vi "Teleop.vi"(10 "Match Info":T1={"Autonomous Elapsed Seconds"=0.0, "TeleOp Elapsed Seconds"=0.0, "Disabled Elapsed Seconds"=0.0, "Visited Autonomous"=FALSE, "Visited TeleOp"=FALSE, "Visited Disabled"=FALSE, "Autonomous Settings"={"Autonomous Style"=enum."Independent", "VI Refnum"=refnum}}, 11 "Call Context":T2) -> ()   [LabVIEW 2019]
doc: "This VI is called for each TeleOp packet received from the DS where the robot is not disabled. It is often used to read from the joysticks and update I/O or to update setpoints for timed control loops. It should complete and return within 20 milliseconds or it may miss DS packets."
uses:
  <vilib>/Rock Robotics/WPI/DriverStation/WPI_DriverStationDerivedRobotMode.ctl
  <vilib>/Rock Robotics/WPI/DriverStation/WPI_DriverStationMatch Info.ctl
  <vilib>/Rock Robotics/WPI/Solenoid/WPI_SolenoidValue.ctl
  <vilib>/Rock Robotics/WPI/ThirdParty/Phoenix-LabVIEW/Motor Controller/Controls/CTRE_Phoenix_MotorControl_ControlMode.ctl
  f70f45e1-7626-4a9c-a34c-83f61dc48ac5.vi
  <vilib>/Rock Robotics/WPI/Utilities/WPI_GetSetVariantRefNum.vi
  <vilib>/Rock Robotics/Network Tables/NT Write Boolean Array.vi
  <vilib>/Rock Robotics/Network Tables/NT Write Numeric Array.vi
  <vilib>/Rock Robotics/Network Tables/NT Read Boolean.vi
  <vilib>/Rock Robotics/Network Tables/NT Read Number.vi
  <vilib>/Rock Robotics/WPI/Solenoid/WPI_SolenoidSetEnum.vi
  <vilib>/Rock Robotics/Network Tables/NT Write Boolean.vi
panel:
  out "Sample Slider 0":dbl(slide) scale=0.0..5.0
  out "Sample Boolean 1":bool
  out "Sample Boolean 0":bool
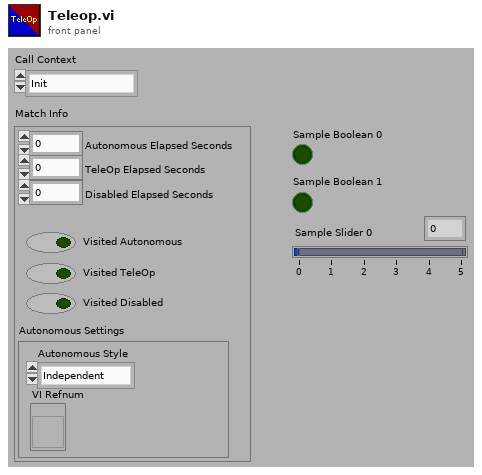
[diagram p1: front panel]
types:
  T1 = typedef "WPI_DriverStationMatch Info.ctl" = cluster{"Autonomous Elapsed Seconds":dbl, "TeleOp Elapsed Seconds":dbl, "Disabled Elapsed Seconds":dbl, "Visited Autonomous":bool, "Visited TeleOp":bool, "Visited Disabled":bool, "Autonomous Settings":cluster{"Autonomous Style":enum16{"Iterative", "Independent"}, "VI Refnum":refnum<vi>}}
  T2 = typedef "WPI_DriverStationDerivedRobotMode.ctl" = enum16{"Init", "Execute", "Stop"}
  T3 = typedef "CTRE_Phoenix_MotorControl_ControlMode.ctl" = u16
  T4 = typedef "WPI_SolenoidValue.ctl" = enum16{"Off", "On", "Forward", "Reverse"}
  T5 = typedef "WPI_JoystickDevRef.ctl" = cluster{"Device":T6}
  T6 = typedef "WPI_JoystickDeviceEnum.ctl" = enum16{"USB 0", "USB 1", "USB 2", "USB 3", "USB 4", "USB 5"}
  T7 = typedef "WPI_RobotDriveDevRef.ctl" = cluster{"DevStatus":errorcluster, "Motors[]":T8[], "Square Inputs":bool, "Max Output":dbl}
  T8 = typedef "WPI_MotorControlDeviceRef.ctl" = cluster{"DeviceStatus":errorcluster, "Type":T9, "PWM":cluster{"PWM Channel":T10, "DeadBand":T11}, "CAN":cluster{"Device Number":u8, "SetOutput VI Ref":variant, "GetOutput VI Ref":variant, "Enable VI Ref":variant, "Disable VI Ref":variant, "Data":variant}, "Invert":bool, "DIO PWM":cluster{"PWM \"Enable\" Channel":T10, "DIOChannel":T12, "PWM Rate":dbl}}
  T9 = typedef "WPI_MotorControlType.ctl" = enum16{"PWM", "CAN", "DIO PWM"}
  T10 = typedef "FPGA_DIOPWMChannel.ctl" = enum8{"PWM 0", "PWM 1", "PWM 2", "PWM 3", "PWM 4", "PWM 5", "PWM 6", "PWM 7", "PWM 8", "PWM 9", "PWM MXP 0", "PWM MXP 1", "PWM MXP 2", "PWM MXP 3", "PWM MXP 4", "PWM MXP 5", "PWM MXP 6", "PWM MXP 7", "PWM MXP 8", "PWM MXP 9", "Invalid"}
  T11 = typedef "WPI_PWMDeadband.ctl" = cluster{"Name":string, "maxPositivePwm":i32, "minPositivePwm":i32, "centerPwm":i32, "maxNegativePwm":i32, "minNegativePwm":i32, "angularRange":u16}
  T12 = typedef "FPGA_DIOChannel.ctl" = enum8{"DIO 0", "DIO 1", "DIO 2", "DIO 3", "DIO 4", "DIO 5", "DIO 6", "DIO 7", "DIO 8", "DIO 9", "DIO MXP 0", "DIO MXP 1", "DIO MXP 2", "DIO MXP 3", "DIO MXP 4", "DIO MXP 5", "DIO MXP 6", "DIO MXP 7", "DIO MXP 8", "DIO MXP 9", "DIO MXP 10", "DIO MXP 11", "DIO MXP 12", "DIO MXP 13", "DIO MXP 14", "DIO MXP 15", "SPI Port CS1", "SPI Port CS2", "SPI Port CS3", "SPI Port MISO", "SPI Port MOSI", "Invalid"}
  T13 = typedef "WPI_SolenoidDevRef.ctl" = cluster{"DevStatus":errorcluster, "Pneumatics Control Module":u8, "Forward Solenoid Channel":T14, "Reverse Solenoid Channel":T14}
  T14 = typedef "WPI_SolenoidChannel.ctl" = enum8{"Solenoid 0", "Solenoid 1", "Solenoid 2", "Solenoid 3", "Solenoid 4", "Solenoid 5", "Solenoid 6", "Solenoid 7", "Invalid"}
  T15 = typedef "WPI_DigitalInputDevRef.ctl" = cluster{"DevStatus":errorcluster, "DIO Channel":T12}
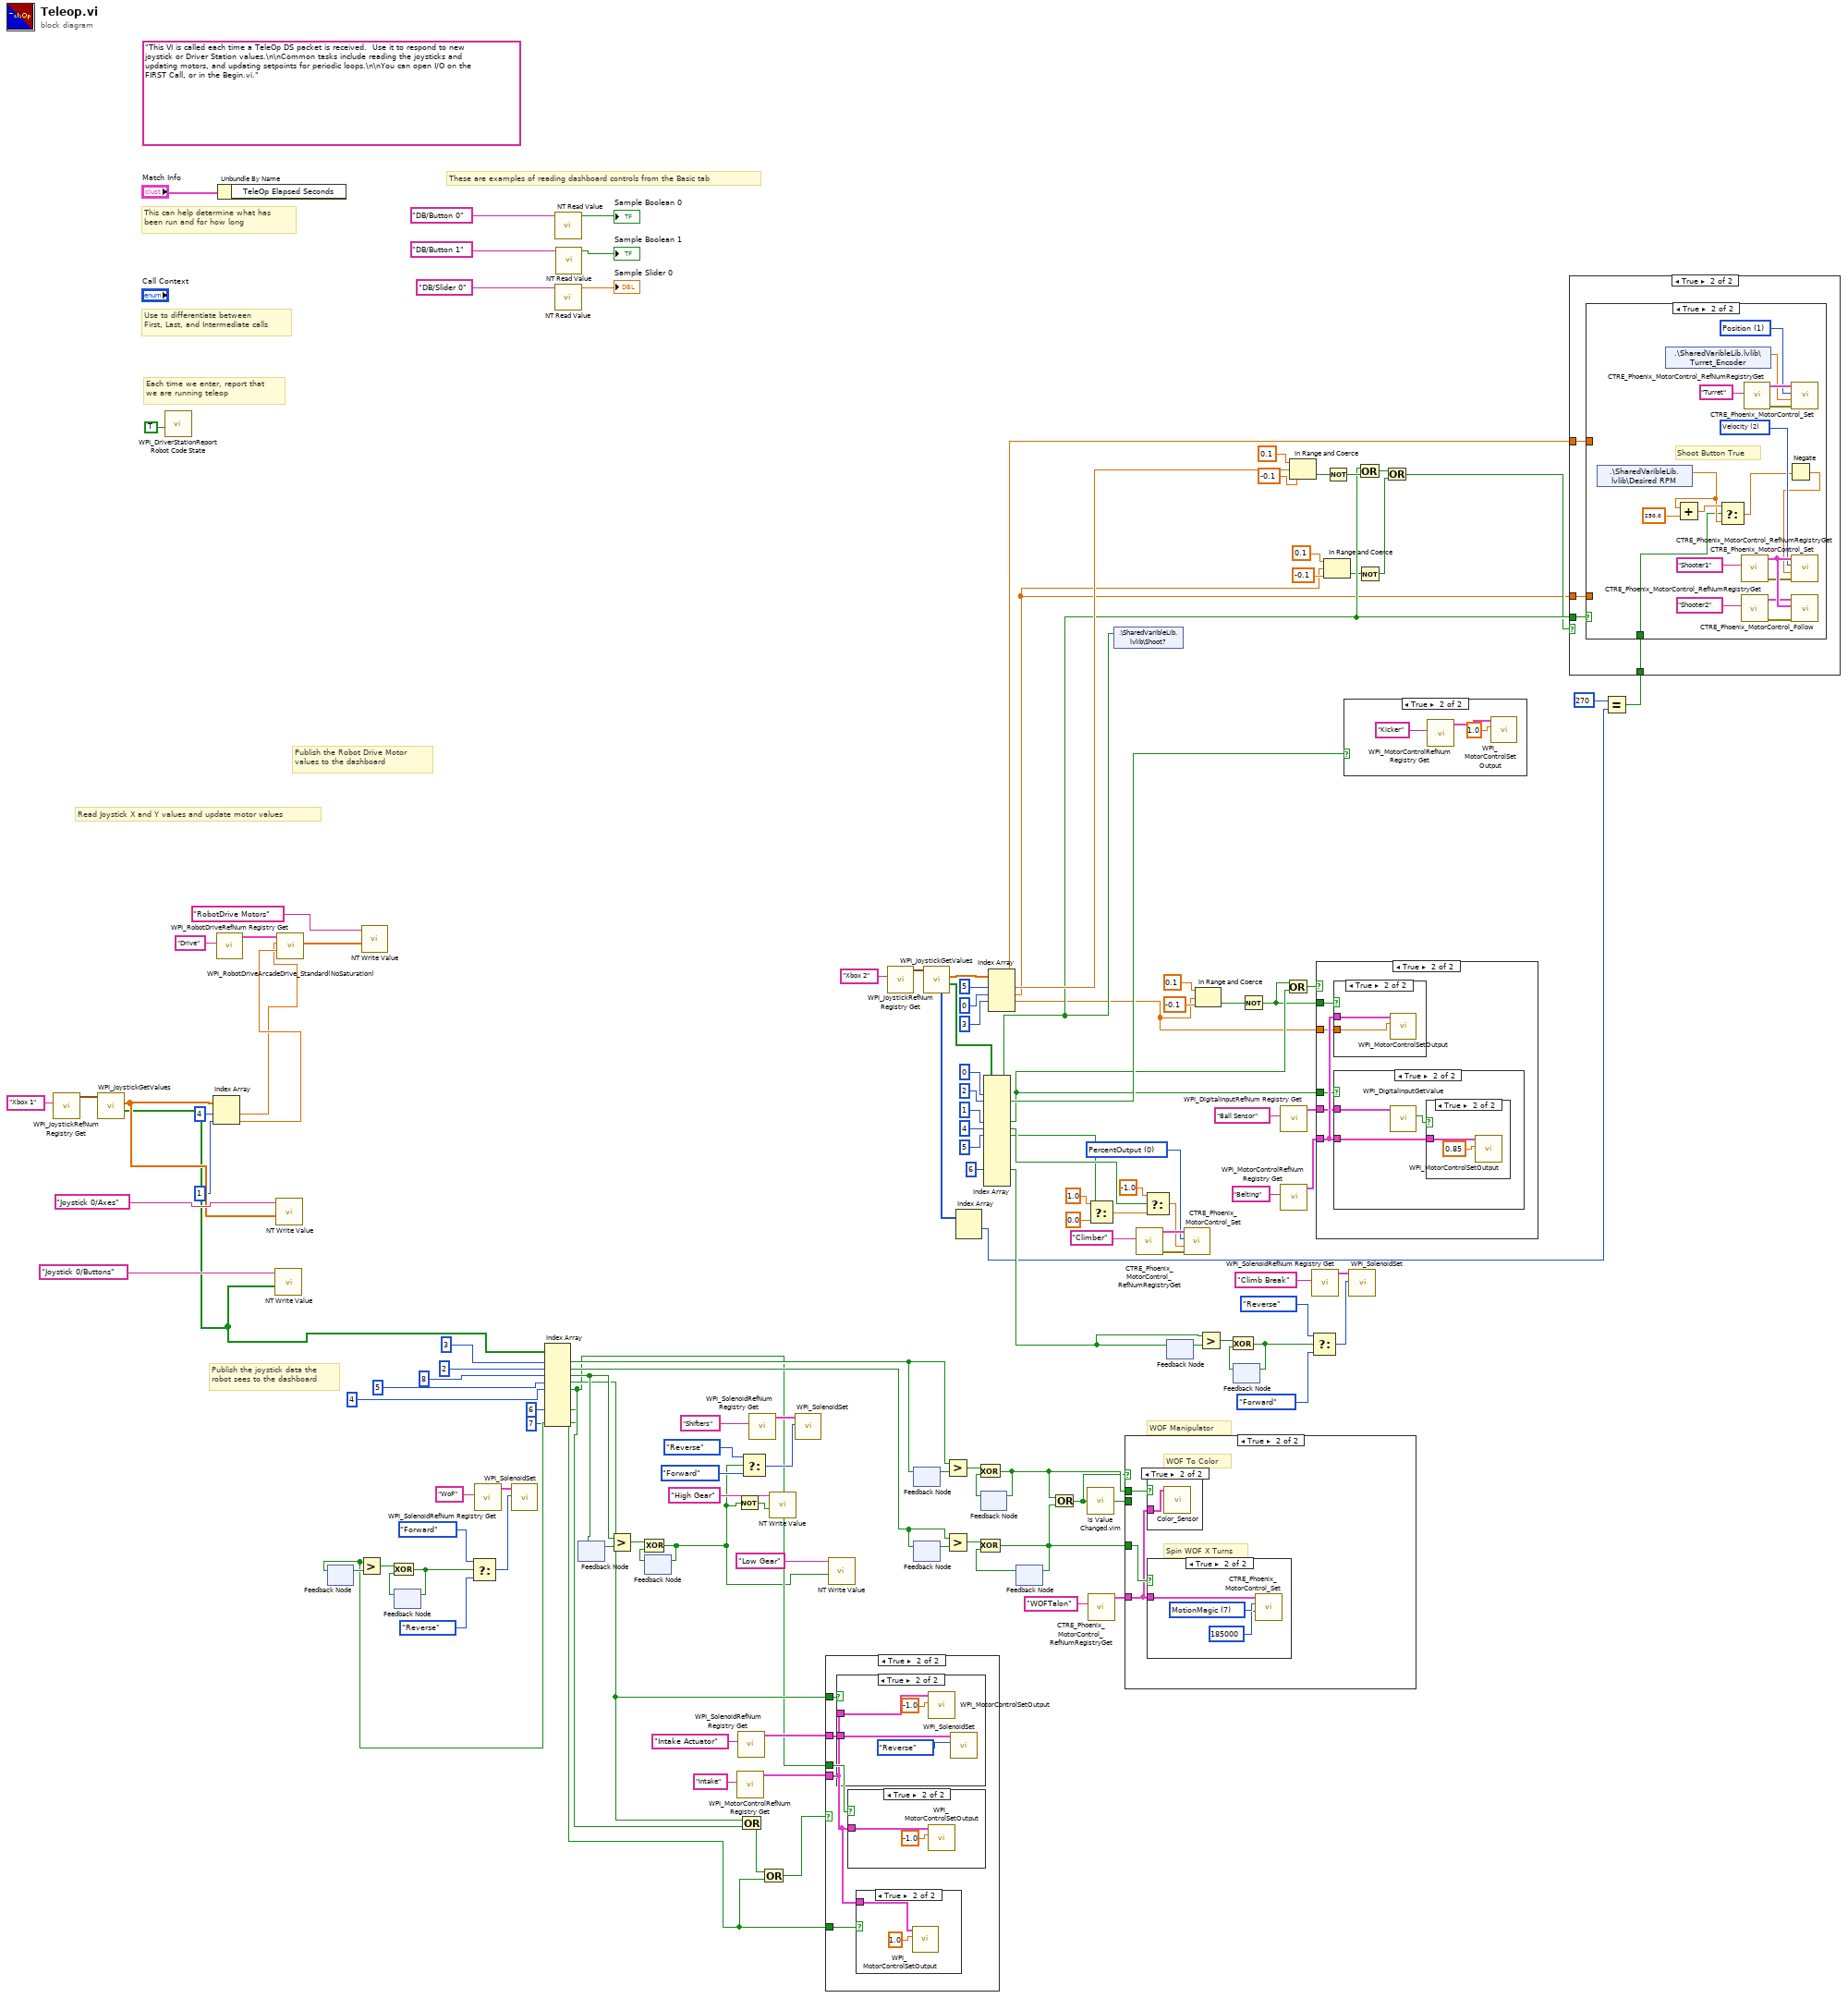
[diagram p0: block diagram]
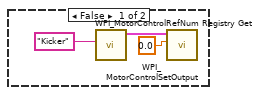
[diagram p2: hidden frame]
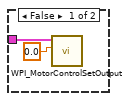
[diagram p3: hidden frame]
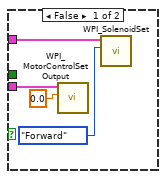
[diagram p7: hidden frame]
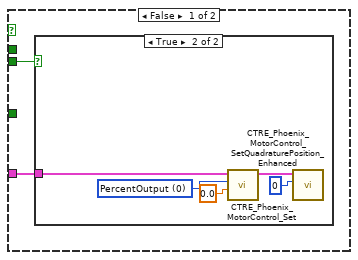
[diagram p11: hidden frame]
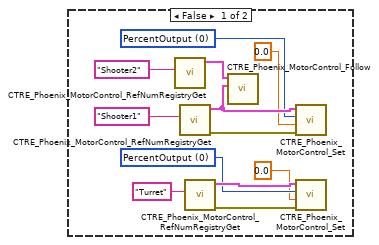
[diagram p15: hidden frame]
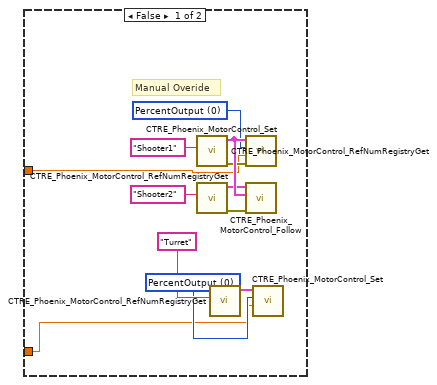
[diagram p16: hidden frame]
diagram:
  w8 = T3 0 items=["PercentOutput"=0, "Position"=1, "Velocity"=2, "Current"=3, "Follower"=5, "MotionProfile"=6, "MotionMagic"=7, "MotionProfileArc"=10, "Disabled"=15] ("Control Mode")
  (unwired) "This VI is called each time a TeleOp DS packet is received.  Use it to respond to new joystick or Driver Station values.\n\nCommon tasks include reading the joysticks and updating motors, and updating setpoints for periodic loops.\n\nYou can open I/O on the FIRST Call, or in the Begin.vi."
  # "WOF Manipulator"
  # "These are examples of reading dashboard controls from the Basic tab"
  # "Publish the Robot Drive Motor\nvalues to the dashboard"
  # "Publish the joystick data the\nrobot sees to the dashboard"
  # "Each time we enter, report that\nwe are running teleop"
  # "Use to differentiate between\nFirst, Last, and Intermediate calls"
  # "This can help determine what has\nbeen run and for how long"
  # "Read Joystick X and Y values and update motor values"
  n1 = call <vilib>:"WPI_JoystickRefNum Registry Get.vi"("refnum name"="Xbox 1") -> ("JoystickDevRef"=w136:T5)  [unwired: 1 in, 9 out]
  n2 = call <vilib>:"WPI_JoystickGetValues.vi"("JoystickDevRef"=w136) -> ("Buttons"=w123:bool[], "Axes"=w132:dbl[])  [unwired: 6 in, 3 out]
  n3 = call <vilib>:"WPI_DriverStationReport Robot Code State.vi"("TeleOp"=TRUE ("Autonomous")) -> ()  [unwired: 10 in, 1 out]
  n4 = Index Array(array=w132, index #1=4 ("index"), index #2=1 ("index")) -> (element #1=w60:dbl, element #2=w61:dbl)
  n5 = call <vilib>:"WPI_RobotDriveRefNum Registry Get.vi"("refnum name"="Drive") -> ("RobotDriveDevRef"=w45:T7)  [unwired: 1 in, 9 out]
  n6 = Unbundle By Name("Match Info") -> ()  [unwired: 1 out]
  n7 = call-poly <vilib>:"NT Write Value.vi"("Boolean Array"=w123, "Name"="Joystick 0/Buttons") -> ()  [unwired: 9 in, 1 out]
  n8 = call-poly <vilib>:"NT Write Value.vi"("Numeric Array"=w132, "Name"="Joystick 0/Axes") -> ()  [unwired: 9 in, 1 out]
  n9 = call <vilib>:"WPI_RobotDriveArcadeDrive_Standard(NoSaturation).vi"("Y axis value"=w61, "X axis value"=w60, "RobotDriveDevRef"=w45) -> ("Motor Values"=w44:dbl[])  [unwired: 1 in, 7 out]
  n10 = feedback #1() -> (w51:bool)  [unwired: 1 in]
  n11 = call-poly <vilib>:"NT Write Value.vi"("Numeric Array"=w44, "Name"="RobotDrive Motors") -> ()  [unwired: 9 in, 1 out]
  n12 = feedback #2() -> (w49:bool)  [unwired: 1 in]
  n13 = call <vilib>:"WPI_SolenoidRefNum Registry Get.vi"("refnum name"="WoF") -> ("SolenoidDevRef"=w52:T13)  [unwired: 9 in, 1 out]
  n14 = Index Array(array=w123, index #1=3 ("index"), index #2=2 ("index"), index #3=8 ("index"), index #4=5 ("index"), index #5=4 ("index"), index #8=6 ("index"), index #10=7 ("index")) -> (element #1=w119:bool, element #2=w118:bool, element #3=w107:bool, element #4=w59:bool, element #5=w57:bool, element #8=w47:bool, element #10=w18:bool)  [unwired: 3 in, 3 out]
  n15 = feedback-in #1(w47) -> ()
  n16 = Greater?(x=w47, y=w51) -> (0:w50:bool)
  n17 = Exclusive Or(1:w49, 2:w50) -> (0:w48:bool)
  n18 = feedback-in #2(w48) -> ()
  n19 = Select(t=WPI_SolenoidValue."Forward" ("Value"), s=w48, f=WPI_SolenoidValue."Reverse" ("Value")) -> (s? t:f=w54:T4)
  n20 = call-poly <vilib>:"WPI_SolenoidSet.vi"("Value"=w54, "SolenoidDevRef"=w52) -> ()  [unwired: 8 in, 2 out]
  n21 = call-poly <vilib>:"NT Read Value.vi"("Name"="DB/Button 0" ("refnum name")) -> ("Boolean"=→"Sample Boolean 0":bool)  [unwired: 9 in, 1 out]
  n22 = call-poly <vilib>:"NT Read Value.vi"("Name"="DB/Slider 0" ("refnum name")) -> ("Numeric"=→"Sample Slider 0":dbl)  [unwired: 9 in, 1 out]
  n23 = call-poly <vilib>:"NT Read Value.vi"("Name"="DB/Button 1" ("refnum name")) -> ("Boolean"=→"Sample Boolean 1":bool)  [unwired: 9 in, 1 out]
  n24 = feedback #3() -> (w117:bool)  [unwired: 1 in]
  n25 = feedback-in #3(w107) -> ()
  n26 = Greater?(x=w107, y=w117) -> (0:w116:bool)
  n27 = feedback #4() -> (w115:bool)  [unwired: 1 in]
  n28 = Exclusive Or(1:w115, 2:w116) -> (0:w5:bool)
  n29 = feedback-in #4(w5) -> ()
  n30 = Not(x=w5) -> (.not. x?=w6:bool)
  n31 = call <vilib>:"WPI_MotorControlRefNum Registry Get.vi"("refnum name"="Intake") -> ("MotorControlDevRef"=w68:T8)  [unwired: 9 in, 1 out]
  n32 = call <vilib>:"WPI_SolenoidRefNum Registry Get.vi"("refnum name"="Intake Actuator") -> ("SolenoidDevRef"=w66:T13)  [unwired: 9 in, 1 out]
  n33 = Or(x=w59, y=w57) -> (x .or. y?=w17:bool)
  n34 = Select(t=WPI_SolenoidValue."Reverse" ("Value"), s=w5, f=WPI_SolenoidValue."Forward" ("Value")) -> (s? t:f=w112:T4)
  n35 = call <vilib>:"WPI_SolenoidRefNum Registry Get.vi"("refnum name"="Shifters") -> ("SolenoidDevRef"=w110:T13)  [unwired: 9 in, 1 out]
  n36 = Or(x=w17, y=w18) -> (x .or. y?=w16:bool)
  n37 = call-poly <vilib>:"NT Write Value.vi"("Boolean"=w6, "Name"="High Gear") -> ()  [unwired: 9 in, 1 out]
  n38 = call-poly <vilib>:"WPI_SolenoidSet.vi"("Value"=w112, "SolenoidDevRef"=w110) -> ()  [unwired: 8 in, 2 out]
  n39 = case shown="True" w16 {
    tunnel: w59 -> [_ w147]
    tunnel: w57 -> [_ w146]
    tunnel: w68 -> [w140 w144]
    tunnel: w66 -> [w139 w145]
    tunnel: w18 -> [_ w143]
    frame False {
      n40 = call <vilib>:"WPI_MotorControlSetOutput.vi"("Output"=0.0, "MotorControlDevRef"=w140) -> ()  [unwired: 7 in, 3 out]
      n41 = call-poly <vilib>:"WPI_SolenoidSet.vi"("Value"=WPI_SolenoidValue."Forward", "SolenoidDevRef"=w139) -> ()  [unwired: 8 in, 2 out]
    }
    frame True {
      n42 = case shown="True" w147 {
        tunnel: w144 -> [_ w154]
        tunnel: w145 -> [_ w153]
        frame False {
        }
        frame True {
          n43 = call <vilib>:"WPI_MotorControlSetOutput.vi"("Output"=-1.0, "MotorControlDevRef"=w154) -> ()  [unwired: 7 in, 3 out]
          n44 = call-poly <vilib>:"WPI_SolenoidSet.vi"("Value"=WPI_SolenoidValue."Reverse", "SolenoidDevRef"=w153) -> ()  [unwired: 8 in, 2 out]
        }
      }
      n45 = case shown="True" w146 {
        tunnel: w144 -> [_ w150]
        frame False {
        }
        frame True {
          n46 = call <vilib>:"WPI_MotorControlSetOutput.vi"("Output"=-1.0, "MotorControlDevRef"=w150) -> ()  [unwired: 7 in, 3 out]
        }
      }
      n47 = case shown="True" w143 {
        tunnel: w144 -> [_ w148]
        frame False {
        }
        frame True {
          n48 = call <vilib>:"WPI_MotorControlSetOutput.vi"("Output"=1.0, "MotorControlDevRef"=w148) -> ()  [unwired: 7 in, 3 out]
        }
      }
    }
  }
  n49 = call-poly <vilib>:"NT Write Value.vi"("Boolean"=w5, "Name"="Low Gear") -> ()  [unwired: 9 in, 1 out]
  n50 = call <vilib>:"WPI_JoystickRefNum Registry Get.vi"("refnum name"="Xbox 2") -> ("JoystickDevRef"=w105:T5)  [unwired: 1 in, 9 out]
  n51 = feedback #5() -> (w81:bool)  [unwired: 1 in]
  n52 = feedback-in #5(w119) -> ()
  n53 = feedback #6() -> (w77:bool)  [unwired: 1 in]
  n54 = feedback-in #6(w118) -> ()
  n55 = call <vilib>:"WPI_JoystickGetValues.vi"("JoystickDevRef"=w105) -> ("Buttons"=w103:bool[], "Axes"=w104:dbl[], "POVs"=w3:i16[])  [unwired: 6 in, 2 out]
  n56 = Greater?(x=w119, y=w81) -> (0:w80:bool)
  n57 = Greater?(x=w118, y=w77) -> (0:w76:bool)
  n58 = Index Array(array=w3) -> (element #1=w2:i16)  [unwired: 2 in, 1 out]
  n59 = feedback #7() -> (w79:bool)  [unwired: 1 in]
  n60 = Exclusive Or(1:w79, 2:w80) -> (0:w74:bool)
  n61 = feedback-in #7(w74) -> ()
  n62 = Index Array(array=w103, index #1=0 ("index"), index #2=2 ("index"), index #5=1 ("index"), index #6=4 ("index"), index #7=5 ("index"), index #12=6 ("index")) -> (element #1=w92:bool, element #2=w84:bool, element #5=w38:bool, element #6=w34:bool, element #7=w33:bool, element #12=w22:bool)  [unwired: 8 in, 8 out]
  n63 = Index Array(array=w104, index #1=5 ("index"), index #2=0 ("index"), index #3=3 ("index")) -> (element #1=w93:dbl, element #2=w87:dbl, element #3=w36:dbl)  [unwired: 1 in, 1 out]
  n64 = feedback #8() -> (w75:bool)  [unwired: 1 in]
  n65 = Exclusive Or(1:w75, 2:w76) -> (0:w73:bool)
  n66 = feedback-in #8(w73) -> ()
  n67 = Or(x=w74, y=w73) -> (x .or. y?=w72:bool)
  n68 = call "Is Value Changed.vim"("value"=w72) -> ("changed or first call?"=w71:bool)
  n69 = Select(t=1.0, s=w33, f=0.0) -> (s? t:f=w11:dbl)
  n70 = call <vilib>:"CTRE_Phoenix_MotorControl_RefNumRegistryGet.vi"("refnum name"="WOFTalon") -> ("PhoenixMotorControlDevRef"=w70:T8)  [unwired: 9 in, 1 out]
  n71 = shared-variable ".\\SharedVaribleLib.lvlib\\Shoot?"(w92) -> ()  [unwired: 1 in, 1 out]
  n72 = case shown="True" w72 {
    tunnel: w74 -> [_ w165]
    tunnel: w70 -> [w157 w163]
    tunnel: w73 -> [_ w164]
    tunnel: w71 -> [w156 _]
    frame False {
      n73 = case shown="True" w156 {
        tunnel: w157 -> [_ w160]
        frame False {
        }
        frame True {
          w162 = T3 0 items=["PercentOutput"=0, "Position"=1, "Velocity"=2, "Current"=3, "Follower"=5, "MotionProfile"=6, "MotionMagic"=7, "MotionProfileArc"=10, "Disabled"=15] ("Control Mode")
          n74 = call <vilib>:"CTRE_Phoenix_MotorControl_Set.vi"("Output"=0.0, "Control Mode"=w162, "PhoenixMotorControlDevRef"=w160) -> ("PhoenixMotorControlDevRef"=w158:T8)  [unwired: 7 in, 1 out]
          n75 = call <vilib>:"CTRE_Phoenix_MotorControl_SetQuadraturePosition_Enhanced.vi"("New Position"=0, "PhoenixMotorControlDevRef"=w158) -> ()  [unwired: 8 in, 2 out]
        }
      }
    }
    frame True {
      # "WOF To Color"
      # "Spin WOF X Turns"
      n76 = case shown="True" w165 {
        tunnel: w163 -> [_ w169]
        frame False {
        }
        frame True {
          n77 = call "Color_Sensor.vi"("PhoenixMotorControlDevRef"=w169) -> ()  [unwired: 11 in]
        }
      }
      n78 = case shown="True" w164 {
        tunnel: w163 -> [_ w166]
        frame False {
        }
        frame True {
          w168 = T3 7 items=["PercentOutput"=0, "Position"=1, "Velocity"=2, "Current"=3, "Follower"=5, "MotionProfile"=6, "MotionMagic"=7, "MotionProfileArc"=10, "Disabled"=15] ("Control Mode")
          n79 = call <vilib>:"CTRE_Phoenix_MotorControl_Set.vi"("Output"=185000 ("x"), "Control Mode"=w168, "PhoenixMotorControlDevRef"=w166) -> ()  [unwired: 7 in, 2 out]
        }
      }
    }
  }
  n80 = call <vilib>:"CTRE_Phoenix_MotorControl_RefNumRegistryGet.vi"("refnum name"="Climber") -> ("error out"=w14:errorcluster, "PhoenixMotorControlDevRef"=w15:T8)  [unwired: 9 in]
  n81 = Select(t=-1.0, s=w34, f=w11) -> (s? t:f=w9:dbl)
  n82 = feedback #9() -> (w21:bool)  [unwired: 1 in]
  n83 = feedback-in #9(w22) -> ()
  n84 = call <vilib>:"CTRE_Phoenix_MotorControl_Set.vi"("error in (no error)"=w14, "Output"=w9, "Control Mode"=w8, "PhoenixMotorControlDevRef"=w15) -> ()  [unwired: 6 in, 2 out]
  n85 = In Range and Coerce(upper limit=0.1, x=w36, lower limit=-0.1) -> (In Range?=w40:bool)  [unwired: 1 out]
  n86 = Greater?(x=w22, y=w21) -> (0:w25:bool)
  n87 = feedback #10() -> (w24:bool)  [unwired: 1 in]
  n88 = Exclusive Or(1:w24, 2:w25) -> (0:w23:bool)
  n89 = feedback-in #10(w23) -> ()
  n90 = Not(x=w40) -> (.not. x?=w37:bool)
  n91 = call <vilib>:"WPI_DigitalInputRefNum Registry Get.vi"("refnum name"="Ball Sensor") -> ("DigitalInputDevRef"=w62:T15)  [unwired: 9 in, 1 out]
  n92 = call <vilib>:"WPI_MotorControlRefNum Registry Get.vi"("refnum name"="Belting") -> ("MotorControlDevRef"=w64:T8)  [unwired: 9 in, 1 out]
  n93 = Or(x=w37, y=w38) -> (x .or. y?=w39:bool)
  n94 = In Range and Coerce(upper limit=0.1, x=w93, lower limit=-0.1) -> (In Range?=w101:bool)  [unwired: 1 out]
  n95 = Select(t=WPI_SolenoidValue."Reverse" ("Value"), s=w23, f=WPI_SolenoidValue."Forward" ("Value")) -> (s? t:f=w28:T4)
  n96 = call <vilib>:"WPI_SolenoidRefNum Registry Get.vi"("refnum name"="Climb Break") -> ("SolenoidDevRef"=w26:T13)  [unwired: 9 in, 1 out]
  n97 = case shown="True" w39 {
    tunnel: w64 -> [w170 w176]
    tunnel: w62 -> [_ w175]
    tunnel: w38 -> [_ w174]
    tunnel: w37 -> [_ w173]
    tunnel: w36 -> [_ w172]
    frame False {
      n98 = call <vilib>:"WPI_MotorControlSetOutput.vi"("Output"=0.0, "MotorControlDevRef"=w170) -> ()  [unwired: 7 in, 3 out]
    }
    frame True {
      n99 = case shown="True" w173 {
        tunnel: w176 -> [_ w178]
        tunnel: w172 -> [_ w177]
        frame False {
        }
        frame True {
          n100 = call <vilib>:"WPI_MotorControlSetOutput.vi"("Output"=w177, "MotorControlDevRef"=w178) -> ()  [unwired: 7 in, 3 out]
        }
      }
      n101 = case shown="True" w174 {
        tunnel: w176 -> [_ w180]
        tunnel: w175 -> [_ w179]
        frame False {
        }
        frame True {
          n102 = call <vilib>:"WPI_DigitalInputGetValue.vi"("DigitalInputDevRef"=w179) -> ("Value"=w181:bool)  [unwired: 8 in, 2 out]
          n103 = case shown="True" w181 {
            tunnel: w180 -> [_ w182]
            frame False {
            }
            frame True {
              n104 = call <vilib>:"WPI_MotorControlSetOutput.vi"("Output"=0.85, "MotorControlDevRef"=w182) -> ()  [unwired: 7 in, 3 out]
            }
          }
        }
      }
    }
  }
  n105 = In Range and Coerce(upper limit=0.1, x=w87, lower limit=-0.1) -> (In Range?=w91:bool)  [unwired: 1 out]
  n106 = Not(x=w101) -> (.not. x?=w100:bool)
  n107 = case shown="True" w84 {
    frame False {
      n108 = call <vilib>:"WPI_MotorControlRefNum Registry Get.vi"("refnum name"="Kicker") -> ("MotorControlDevRef"=w186:T8)  [unwired: 9 in, 1 out]
      n109 = call <vilib>:"WPI_MotorControlSetOutput.vi"("Output"=0.0, "MotorControlDevRef"=w186) -> ()  [unwired: 7 in, 3 out]
    }
    frame True {
      n110 = call <vilib>:"WPI_MotorControlRefNum Registry Get.vi"("refnum name"="Kicker") -> ("MotorControlDevRef"=w189:T8)  [unwired: 9 in, 1 out]
      n111 = call <vilib>:"WPI_MotorControlSetOutput.vi"("Output"=1.0, "MotorControlDevRef"=w189) -> ()  [unwired: 7 in, 3 out]
    }
  }
  n112 = call-poly <vilib>:"WPI_SolenoidSet.vi"("Value"=w28, "SolenoidDevRef"=w26) -> ()  [unwired: 8 in, 2 out]
  n113 = Or(x=w92, y=w100) -> (x .or. y?=w90:bool)
  n114 = Not(x=w91) -> (.not. x?=w89:bool)
  n115 = Or(x=w90, y=w89) -> (x .or. y?=w88:bool)
  n116 = Equal?(x=i16 270, y=w2) -> (x = y?=w4:bool)
  n117 = case shown="True" w88 {
    tunnel: w93 -> [_ w205]
    tunnel: w92 -> [_ w204]
    tunnel: w87 -> [_ w203]
    tunnel: w4 -> [_ w202]
    frame False {
      w191 = T3 0 items=["PercentOutput"=0, "Position"=1, "Velocity"=2, "Current"=3, "Follower"=5, "MotionProfile"=6, "MotionMagic"=7, "MotionProfileArc"=10, "Disabled"=15] ("Control Mode")
      w198 = T3 0 items=["PercentOutput"=0, "Position"=1, "Velocity"=2, "Current"=3, "Follower"=5, "MotionProfile"=6, "MotionMagic"=7, "MotionProfileArc"=10, "Disabled"=15] ("Control Mode")
      n118 = call <vilib>:"CTRE_Phoenix_MotorControl_RefNumRegistryGet.vi"("refnum name"="Shooter2") -> ("PhoenixMotorControlDevRef"=w199:T8)  [unwired: 9 in, 1 out]
      n119 = call <vilib>:"CTRE_Phoenix_MotorControl_RefNumRegistryGet.vi"("refnum name"="Shooter1") -> ("error out"=w197:errorcluster, "PhoenixMotorControlDevRef"=w201:T8)  [unwired: 9 in]
      n120 = call <vilib>:"CTRE_Phoenix_MotorControl_RefNumRegistryGet.vi"("refnum name"="Turret") -> ("error out"=w193:errorcluster, "PhoenixMotorControlDevRef"=w194:T8)  [unwired: 9 in]
      n121 = call <vilib>:"CTRE_Phoenix_MotorControl_Follow.vi"("Master Controller to Follow"=w201, "PhoenixMotorControlDevRef"=w199) -> ()  [unwired: 8 in, 2 out]
      n122 = call <vilib>:"CTRE_Phoenix_MotorControl_Set.vi"("error in (no error)"=w197, "Output"=0.0 ("upper limit"), "Control Mode"=w198, "PhoenixMotorControlDevRef"=w201) -> ()  [unwired: 6 in, 2 out]
      n123 = call <vilib>:"CTRE_Phoenix_MotorControl_Set.vi"("error in (no error)"=w193, "Output"=0.0, "Control Mode"=w191, "PhoenixMotorControlDevRef"=w194) -> ()  [unwired: 6 in, 2 out]
    }
    frame True {
      n124 = case shown="True" w204 {
        tunnel: w205 -> [w210 _]
        tunnel: w203 -> [w206 _]
        tunnel: w202 -> [_ w218]
        frame False {
          w207 = T3 0 items=["PercentOutput"=0, "Position"=1, "Velocity"=2, "Current"=3, "Follower"=5, "MotionProfile"=6, "MotionMagic"=7, "MotionProfileArc"=10, "Disabled"=15] ("Control Mode")
          w213 = T3 0 items=["PercentOutput"=0, "Position"=1, "Velocity"=2, "Current"=3, "Follower"=5, "MotionProfile"=6, "MotionMagic"=7, "MotionProfileArc"=10, "Disabled"=15] ("Control Mode")
          # "Manual Overide"
          n125 = call <vilib>:"CTRE_Phoenix_MotorControl_RefNumRegistryGet.vi"("refnum name"="Shooter1") -> ("error out"=w212:errorcluster, "PhoenixMotorControlDevRef"=w217:T8)  [unwired: 9 in]
          n126 = call <vilib>:"CTRE_Phoenix_MotorControl_RefNumRegistryGet.vi"("refnum name"="Shooter2") -> ("error out"=w215:errorcluster, "PhoenixMotorControlDevRef"=w214:T8)  [unwired: 9 in]
          n127 = call <vilib>:"CTRE_Phoenix_MotorControl_RefNumRegistryGet.vi"("refnum name"="Turret") -> ("PhoenixMotorControlDevRef"=w209:T8)  [unwired: 9 in, 1 out]
          n128 = call <vilib>:"CTRE_Phoenix_MotorControl_Set.vi"("error in (no error)"=w212, "Output"=w210, "Control Mode"=w213, "PhoenixMotorControlDevRef"=w217) -> ()  [unwired: 6 in, 2 out]
          n129 = call <vilib>:"CTRE_Phoenix_MotorControl_Follow.vi"("error in (no error)"=w215, "Master Controller to Follow"=w217, "PhoenixMotorControlDevRef"=w214) -> ()  [unwired: 7 in, 2 out]
          n130 = call <vilib>:"CTRE_Phoenix_MotorControl_Set.vi"("Output"=w206, "Control Mode"=w207, "PhoenixMotorControlDevRef"=w209) -> ()  [unwired: 7 in, 2 out]
        }
        frame True {
          w226 = T3 1 items=["PercentOutput"=0, "Position"=1, "Velocity"=2, "Current"=3, "Follower"=5, "MotionProfile"=6, "MotionMagic"=7, "MotionProfileArc"=10, "Disabled"=15] ("Control Mode")
          w231 = T3 2 items=["PercentOutput"=0, "Position"=1, "Velocity"=2, "Current"=3, "Follower"=5, "MotionProfile"=6, "MotionMagic"=7, "MotionProfileArc"=10, "Disabled"=15] ("Control Mode")
          # "Shoot Button True"
          n131 = shared-variable ".\\SharedVaribleLib.lvlib\\Desired RPM"() -> (w219:dbl)  [unwired: 1 in, 1 out]
          n132 = shared-variable ".\\SharedVaribleLib.lvlib\\Turret_Encoder"() -> (w225:dbl)  [unwired: 1 in, 1 out]
          n133 = Add(x=w219, y=250.0) -> (x+y=w221:dbl)
          n134 = Select(t=w221, s=w218, f=w219) -> (s? t:f=w222:dbl)
          n135 = call <vilib>:"CTRE_Phoenix_MotorControl_RefNumRegistryGet.vi"("refnum name"="Shooter1") -> ("error out"=w230:errorcluster, "PhoenixMotorControlDevRef"=w235:T8)  [unwired: 9 in]
          n136 = call <vilib>:"CTRE_Phoenix_MotorControl_RefNumRegistryGet.vi"("refnum name"="Shooter2") -> ("error out"=w233:errorcluster, "PhoenixMotorControlDevRef"=w232:T8)  [unwired: 9 in]
          n137 = call <vilib>:"CTRE_Phoenix_MotorControl_RefNumRegistryGet.vi"("refnum name"="Turret") -> ("error out"=w228:errorcluster, "PhoenixMotorControlDevRef"=w229:T8)  [unwired: 9 in]
          n138 = Negate(x=w222) -> (-x=w224:dbl)
          n139 = call <vilib>:"CTRE_Phoenix_MotorControl_Set.vi"("error in (no error)"=w228, "Output"=w225, "Control Mode"=w226, "PhoenixMotorControlDevRef"=w229) -> ()  [unwired: 6 in, 2 out]
          n140 = call <vilib>:"CTRE_Phoenix_MotorControl_Set.vi"("error in (no error)"=w230, "Output"=w224, "Control Mode"=w231, "PhoenixMotorControlDevRef"=w235) -> ()  [unwired: 6 in, 2 out]
          n141 = call <vilib>:"CTRE_Phoenix_MotorControl_Follow.vi"("error in (no error)"=w233, "Master Controller to Follow"=w235, "PhoenixMotorControlDevRef"=w232) -> ()  [unwired: 7 in, 2 out]
        }
      }
    }
  }
